vi "PH_Sequencer.SCR Stand by.vi"(0 "i ref in":refnum<vi>, 5 "error in (no error)":errorcluster) -> (14 "i ref out":refnum<vi>, 19 "error out":errorcluster)   [LabVIEW 2014, in "PH_Sequencer.lvlib"]
doc: "This VI sends a state change request to the Seq SM. If the sequencer is in state \"Enable Data Acquisition\", and all PPMA PUs which are use are in PU SM state \"CloseDump Rods\", and all PPPA PUs which are in use are in PU SM state \"Stand by\" or \"Switch PU on\" or \"Set Settings\" or \"Wait for Shot Comd\" or \"Close Ross Relais\", \"Stand by\" is requested."
uses:
  PH_Sequencer.lvlib
  PH_PP_Common/PH_PP_Common.PUs.ctl
  PH_PowerUnit_BaseClass/PH_PowerUnit_BaseClass.SM States.ctl
  CSCore/BaseSM/BaseSM.lvlib
  PH_BeamlineInformation/PH_BeamlineInformation.lvlib
  PH_PP_Common/PH_PP_Common.lvlib
  PH_PowerUnit_BaseClass/PH_PowerUnit_BaseClass.lvlib
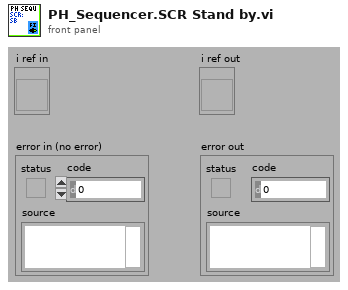
[diagram p1: front panel]
types:
  T1 = typedef "PH_PowerUnit_BaseClass.lvlib/PH_PowerUnit_BaseClass.SM States.ctl" = enum16{".", "Stand by", "Switch PU on", "Configure", "Set Default Voltage", "Set STANDBY", "Set READY", "Wait for Shot Cmd", "Open Dump Rods", "Open Ross Relais", "Close Ross Relais", "Switch PSU on", "Switch PSU off", "Charge", "Switch GD Channel on", "Close Dump Rods", "Rods-TO", "RR-TO", "PSU-TO", "Trigger-TO"}
  T2 = typedef "PH_PP_Common.lvlib/PH_PP_Common.PUs.ctl" = enum16{"no Info", "PA-19mm-1", "PA-19mm-2", "PA-45mm-PILC", "PA-45mm-MAIN", "MA-PU-1", "MA-PU-2", "MA-PU-3", "MA-PU-4", "MA-PU-5", "MA-PU-6", "MA-FR", "MA-PILC", "PA-45mm-DP"}
  T3 = typedef "PH_BeamlineInformation.lvlib/PH_BeamlineInformation.i attribute.ctl" = cluster{"BL GUI Elements of Services":cluster{"Service Name":string, "GUI Elements":refnum<vi>[], "Status":i32}[], "Powermeters":T4, "Efficiency":T5, "Heads":T6[]}
  T4 = typedef "PH_BeamlineInformation.lvlib/PH_BeamlineInformation.Powermeter.ctl" = cluster{"ns FE":cluster{"GUI Ref":refnum<vi>, "Value":dbl}, "fs FE":cluster{"GUI Ref":refnum<vi>, "Value":dbl}, "PA":cluster{"GUI Ref":refnum<vi>, "Value":dbl}, "MA":cluster{"GUI Ref":refnum<vi>, "Value":dbl}, "Z6 green":cluster{"GUI Ref":refnum<vi>, "Value":dbl}, "Z6 IR":cluster{"GUI Ref":refnum<vi>, "Value":dbl}, "Z6 COS":cluster{"GUI Ref":refnum<vi>, "Value":dbl}}
  T5 = typedef "PH_BeamlineInformation.lvlib/PH_BeamlineInformation.Efficiency.ctl" = cluster{"PA Gain":cluster{"GUI Ref":refnum<vi>, "Value":dbl}, "MA Gain":cluster{"GUI Ref":refnum<vi>, "Value":dbl}, "Z6 green Conversion":cluster{"GUI Ref":refnum<vi>, "Value":dbl}, "Z6 Comp Losses":cluster{"GUI Ref":refnum<vi>, "Value":dbl}}
  T6 = typedef "PH_BeamlineInformation.lvlib/PH_BeamlineInformation.Head.ctl" = cluster{"PowerUnit":T2, "in use":cluster{"Value":bool, "GUI Ref":refnum<vi>, "linked":bool}, "voltage":cluster{"Value":dbl, "GUI Ref":refnum<vi>, "linked":bool}}
  T7 = typedef "PH_Sequencer.lvlib/PH_Sequencer.i attribute.ctl" = cluster{"GUI Refs":cluster{"Main Off":refnum<vi>, "Fire":refnum<vi>, "Status":refnum<vi>, "Ready":refnum<vi>, "Waiting Time":refnum<vi>, "Timeout":refnum<vi>, "PPMA Ready":refnum<vi>, "Sequencer SM State":refnum<vi>, "PPPA Ready":refnum<vi>, "Calorimeter":refnum<vi>, "Beamline Ready":refnum<vi>, "Clear Beamline":refnum<vi>, "Linkage PPMA Rods":refnum<vi>, "Linkage Current PA":refnum<vi>, "Linkage Current MA":refnum<vi>, "Timing Ready":refnum<vi>, "State Timing":refnum<vi>, "Force Timing":refnum<vi>, "PSDB Shot Comment":refnum<vi>, "State PA Backreflection":refnum<vi>, "Beamline Z6 Ready":refnum<vi>, "Clear Z6 Beamline":refnum<vi>, "Sequence length":refnum<vi>, "Timing Mode":refnum<vi>, "Slow Trigger Settings":refnum<vi>, "Experiment Description":refnum<vi>, "State PSDB":refnum<vi>, "PSDB Ready":refnum<vi>, "Set PSDB Settings":refnum<vi>, "Get PSDB Info":refnum<vi>, "Take Snapshot":refnum<vi>, "Shottype":refnum<vi>, "Experiment":refnum<vi>, "Phase Frontends":refnum<vi>, "PP 45mm PILC in use":refnum<vi>}, "Status Info":cluster{"Machine Status":T8, "WaitingTime":i32, "Timeout":bool}, "Readyness":cluster{"Ready to shot":bool, "PPMA Ready":bool, "PPPA Ready":bool, "BL Ready":bool, "Timing Ready":bool, "BL Z6 Ready":bool, "PSDBReady":bool}, "Instancenames":cluster{"PPMA Rods":string, "PP Current Meas":string, "PH Beamline Chief":string, "PA Backrefl Meas":string, "Z6 Beamline Chief":string}, "Data to read":bool, "Calorimeter":cluster{"Instancename":string, "On":bool, "linked":bool}, "Linkage":cluster{"PPMA Rods":bool, "PP Current Meas":bool, "PHELIX Beamline Chief":bool, "PA Backrefl Meas":bool, "Z6 Beamline Chief":bool}, "Timing":cluster{"Instance":string, "linked":bool, "Status":T8, "Timing Mode":T9, "Slow Trigger Settings":T10, "Info available":cluster{"ext SlowTrigger":bool, "T2":bool, "Mode":bool, "Delay Slow Trigger":bool, "Phase FEs":bool}, "FE Phase":T11}, "Service ID R2S":i32, "PSDB":cluster{"Controller Instance":string, "Controller Status":T8, "Controller linked":bool, "Settings acknowledged":bool, "Current Experiment ID":i16, "Current Shot Type":i16, "Current Comment":string, "Remember Settings":bool, "Write 2 early":bool}, "PSDB Data":cluster{"Main Off?":bool, "Sequence Length":dbl, "Sequence startet":timestamp}, "6P 4Q Positions":cluster{"Instancename":string, "linked":bool, "Position":T12}[], "PUs":T13[]}
  T8 = typedef "PH_StatusHandler.lvlib/PH_StatusHandler.Status.ctl" = i16
  T9 = typedef "PH_Timing.lvlib/PH_Timing.Timing Mode.ctl" = cluster{"T2":i16, "Modeselector":enum32{"10 Hz", "0.5 Hz", "Shot"}}
  T10 = typedef "PH_Timing.lvlib/PH_Timing.Slow Trigger Settings.ctl" = cluster{"Delay":dbl, "externally triggered?":bool}
  T11 = typedef "PH_Timing.lvlib/PH_Timing.Phase FEs.ctl" = cluster{"Phase":dbl}
  T12 = typedef "PH_4_Pos_Selector.lvlib/PH_4_Pos_Selector.Position Selector.ctl" = u16
  T13 = typedef "PH_Sequencer.lvlib/PH_Sequencer.Head.ctl" = cluster{"PowerUnit":T2, "GUI Ref":refnum<vi>, "Information":T14, "linked?":bool, "GUI Ref Current Voltage":refnum<vi>}
  T14 = typedef "PH_Sequencer.lvlib/PH_Sequencer.PU Information.ctl" = cluster{"State":T8, "Waiting Time [s]":dbl, "PU State SM":T1, "PU Timeout SM":T1}
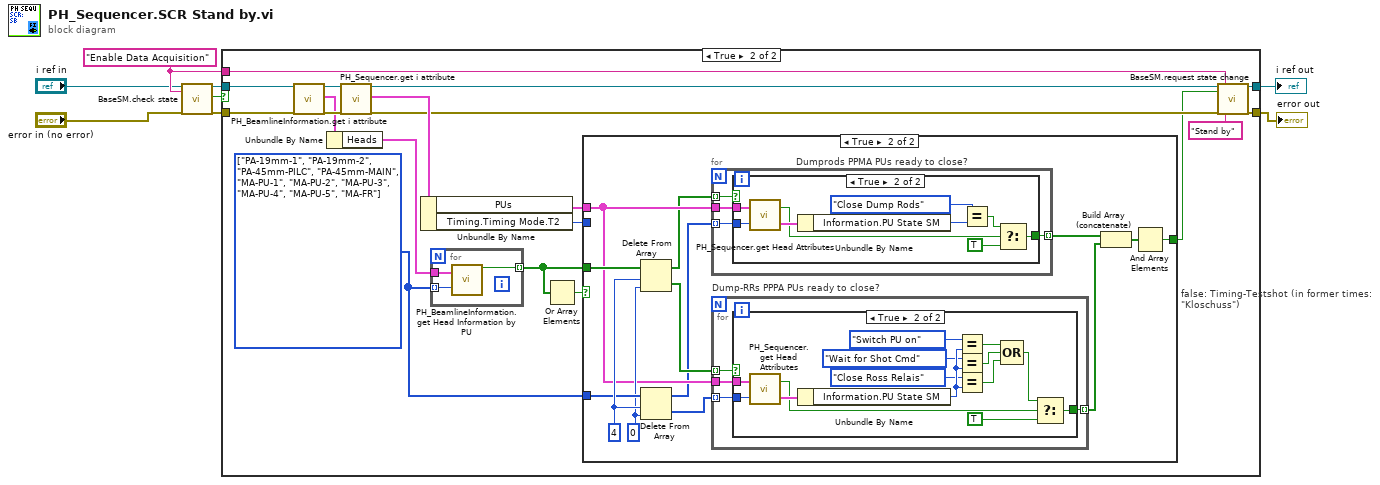
[diagram p0: block diagram]
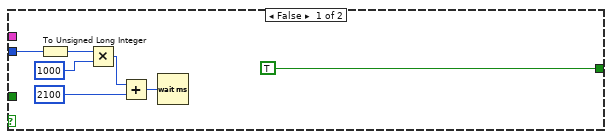
[diagram p3: hidden frame]
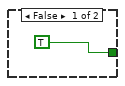
[diagram p4: hidden frame]
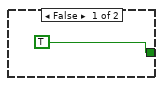
[diagram p5: hidden frame]
diagram:
  w7 = "Enable Data Acquisition" ("requested state")
  n1 = call "BaseSM.check state.vi"("i ref in"="i ref in", "requestedState"=w7, "error in (no error)"="error in (no error)") -> ("i ref out"=w5:refnum<vi>, "OK"=w1:bool, "error out"=w4:errorcluster)  [unwired: 11 in, 3 out]
  n2 = case shown="True" w1 {
    tunnel: [w9 w29] -> w8
    tunnel: w7 -> [_ w28]
    tunnel: [w10 w26] -> w6
    tunnel: w5 -> [w10 w19]
    tunnel: w4 -> [w9 w18]
    frame False {
    }
    frame True {
      w12 = T2[] [enum."PA-19mm-1", enum."PA-19mm-2", enum."PA-45mm-PILC", enum."PA-45mm-MAIN", enum."MA-PU-1", enum."MA-PU-2", enum."MA-PU-3", enum."MA-PU-4", enum."MA-PU-5", enum."MA-FR"] items=["no Info", "PA-19mm-1", "PA-19mm-2", "PA-45mm-PILC", "PA-45mm-MAIN", "MA-PU-1", "MA-PU-2", "MA-PU-3", "MA-PU-4", "MA-PU-5", "MA-PU-6", "MA-FR", "MA-PILC", "PA-45mm-DP"]
      n3 = call "PH_BeamlineInformation.get i attribute.vi"("i ref in"=w19, "error in (no error)"=w18) -> ("i ref out"=w22:refnum<vi>, "i attribute"=w20:T3, "error out"=w23:errorcluster)  [unwired: 15 in]
      n4 = Unbundle By Name(w20) -> ("Heads"=w13:T6[])
      n5 = call "PH_Sequencer.get i attribute.vi"("i ref in"=w22, "error in (no error)"=w23) -> ("i ref out"=w17:refnum<vi>, "i attribute"=w21:T7, "error out"=w16:errorcluster)  [unwired: 15 in]
      n6 = Unbundle By Name(w21) -> ("PUs"=w11:T13[], "Timing.Timing Mode.T2"=w25:i16)
      n7 = for {
        tunnel: [w32] -> w14 mode=indexing
        tunnel: w13 -> [w31]
        tunnel: w12 -> [w30] mode=indexing
        n8 = call "PH_BeamlineInformation.get Head Information by PU.vi"("Heads"=w31, "Power Unit"=w30) -> ("In Use?"=w32:bool)  [unwired: 12 in, 5 out]
      }
      n9 = Or Array Elements(Boolean array=w14) -> (logical OR=w24:bool)
      n10 = case "false: Timing-Testshot (in former times: \"Kloschuss\")" shown="True" w24 {
        tunnel: w14 -> [_ w51]
        tunnel: w25 -> [w34 _]
        tunnel: [TRUE w52] -> w15
        tunnel: w12 -> [_ w45]
        tunnel: w11 -> [_ w43]
        frame False {
          n11 = To Unsigned Long Integer(number=w34) -> (unsigned 32bit integer=w36:u32)
          n12 = Multiply(x=w36, y=u32 1000) -> (x*y=w37:u32)
          n13 = Add(x=w37, y=u32 2100 ("milliseconds to wait")) -> (x+y=w38:u32)
          n14 = Wait (ms)(milliseconds to wait=w38) -> ()  [unwired: 1 out]
        }
        frame True {
          w44 = 0 ("index")
          w46 = 4 ("length")
          n15 = Delete From Array(array=w51, length=w46, index=w44) -> (deleted portion=w48:bool[], array with subset deleted=w42:bool[])
          n16 = Delete From Array(array=w45, length=w46, index=w44) -> (deleted portion=w49:T2[], array with subset deleted=w41:T2[])
          n17 = for "Dumprods PPMA PUs ready to close?" {
            tunnel: [w56] -> w40 mode=indexing
            tunnel: w42 -> [w55] mode=indexing
            tunnel: w41 -> [w54] mode=indexing
            tunnel: w43 -> [w53]
            n18 = case shown="True" w55 {
              tunnel: [TRUE w65] -> w56
              tunnel: w54 -> [_ w63]
              tunnel: w53 -> [_ w64]
              frame False {
              }
              frame True {
                n19 = call "PH_Sequencer.get Head Attributes.vi"("PowerUnit"=w63, "Heads"=w64) -> ("Head"=w62:T13, "Head found?"=w61:bool)
                n20 = Unbundle By Name(w62) -> ("Information.PU State SM"=w60:T1)
                n21 = Equal?(x=PH_PowerUnit_BaseClass.SM_States."Close Dump Rods", y=w60) -> (x = y?=w59:bool)
                n22 = Select(t=w59, s=w61, f=TRUE) -> (s? t:f=w65:bool)
              }
            }
          }
          n23 = for "Dump-RRs PPPA PUs ready to close?" {
            tunnel: [w70] -> w47 mode=indexing
            tunnel: w48 -> [w69] mode=indexing
            tunnel: w49 -> [w68] mode=indexing
            tunnel: w43 -> [w67]
            n24 = case shown="True" w69 {
              tunnel: [TRUE w84] -> w70
              tunnel: w68 -> [_ w82]
              tunnel: w67 -> [_ w83]
              frame False {
              }
              frame True {
                n25 = call "PH_Sequencer.get Head Attributes.vi"("PowerUnit"=w82, "Heads"=w83) -> ("Head"=w81:T13, "Head found?"=w80:bool)
                n26 = Unbundle By Name(w81) -> ("Information.PU State SM"=w79:T1)
                n27 = Equal?(x=PH_PowerUnit_BaseClass.SM_States."Switch PU on", y=w79) -> (x = y?=w78:bool)
                n28 = Equal?(x=PH_PowerUnit_BaseClass.SM_States."Wait for Shot Cmd", y=w79) -> (x = y?=w77:bool)
                n29 = Equal?(x=PH_PowerUnit_BaseClass.SM_States."Close Ross Relais", y=w79) -> (x = y?=w76:bool)
                n30 = Compound Arithmetic op=OR(w78, w77, w76) -> (w75:bool)
                n31 = Select(t=w75, s=w80, f=TRUE) -> (s? t:f=w84:bool)
              }
            }
          }
          n32 = Build Array (concatenate)(w40, w47) -> (w50:bool[])
          n33 = And Array Elements(Boolean array=w50) -> (logical AND=w52:bool)
        }
      }
      n34 = call "BaseSM.request state change.vi"("i ref in"=w17, "change"=w15, "error in (no error)"=w16, "allowed current state"=w28, "requested state"="Stand by" ("next state")) -> ("i ref out"=w26:refnum<vi>, "error out"=w29:errorcluster)  [unwired: 11 in, 2 out]
    }
  }
  "error out" <- w8
  "i ref out" <- w6
